vi "Check endstop str.vi"(8 "error in (no error)":errorcluster, 10 "Ens-stop state in":bool[](array[boolean]), 11 "Data in":string) -> (0 "error out":errorcluster, 2 "Ens-stop state out":bool[](array[boolean]))   [LabVIEW 2020, in "Control de MaP.lvlib"]
uses:
  Control de MaP.lvlib
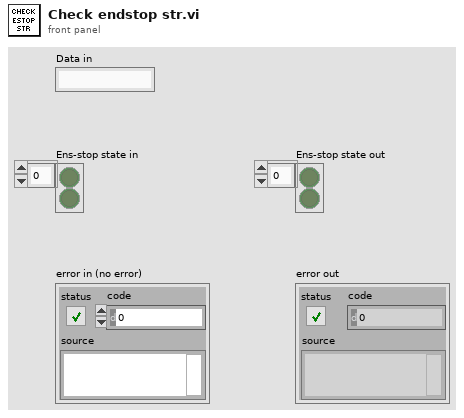
[diagram p1: front panel]
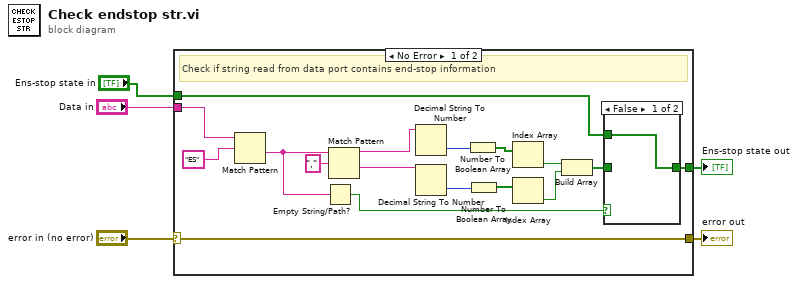
[diagram p0: block diagram]
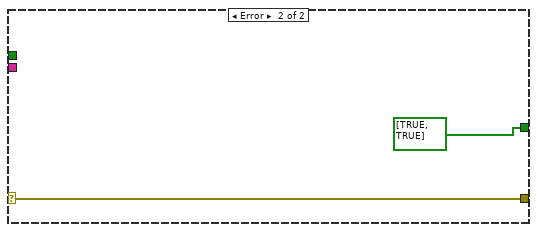
[diagram p3: hidden frame]
diagram:
  n1 = case shown="No Error" "error in (no error)" {
    selector: "error in (no error)" -> [w10 w26]
    tunnel: "Data in" -> [w20 _]
    tunnel: [w7 bool[] [TRUE, TRUE]] -> w4
    tunnel: [w10 w26] -> w2
    tunnel: "Ens-stop state in" -> [w6 _]
    frame No Error {
      # "Check if string read from data port contains end-stop information"
      n2 = Match Pattern(string=w20, regular expression="ES") -> (after substring=w19:string)  [unwired: 1 in, 3 out]
      n3 = Empty String/Path?(string/path=w19) -> (empty?=w9:bool)
      n4 = Match Pattern(string=w19, regular expression=",") -> (before substring=w18:string, after substring=w17:string)  [unwired: 1 in, 2 out]
      n5 = Decimal String To Number(string=w18) -> (number=w16:i32)  [unwired: 2 in, 1 out]
      n6 = Decimal String To Number(string=w17) -> (number=w15:i32)  [unwired: 2 in, 1 out]
      n7 = Number To Boolean Array(number=w16) -> (Boolean array=w14:bool[])
      n8 = Number To Boolean Array(number=w15) -> (Boolean array=w13:bool[])
      n9 = Index Array(array=w14) -> (element=w12:bool)  [unwired: 1 in]
      n10 = Index Array(array=w13) -> (element=w11:bool)  [unwired: 1 in]
      n11 = Build Array(w12, w11) -> (w8:bool[])
      n12 = case shown="False" w9 {
        tunnel: w8 -> [_ w24]
        tunnel: [w23 w24] -> w7
        tunnel: w6 -> [w23 _]
        frame False {
        }
        frame True {
        }
      }
    }
    frame Error {
    }
  }
  "error out" <- w2
  "Ens-stop state out" <- w4
